vi "CreateTableSP.vi"(8 "error in (no error)":errorcluster, 10 "Name of Table":string, 11 "SimulationParameter in":refnum<class "SimulationParameter.lvclass">) -> (0 "error out":errorcluster, 1 "List of Fieldelements":string[](array[string]), 2 "Energy System Setup":string[][](table) caption="Result Set (from first statement with results)", 3 "SimulationParameter out":refnum<class "SimulationParameter.lvclass">)   [LabVIEW 2017, in "SimulationParameter.lvclass"]
uses:
  SimulationParameter.lvclass
  SimulationParameter.lvclass/SimulationParameter.ctl
  <vilib>/drjdpowell/SQLite Library/SQL Connection/Execute SQL (Single Integer).vi
  <vilib>/drjdpowell/SQLite Library/SQL Connection/Execute SQL.vi
  <vilib>/drjdpowell/SQLite Library/SQLite.lvlib
  <vilib>/drjdpowell/SQLite Library/SQL Connection/Connection.lvclass
panel:
  out "concatenated string":string
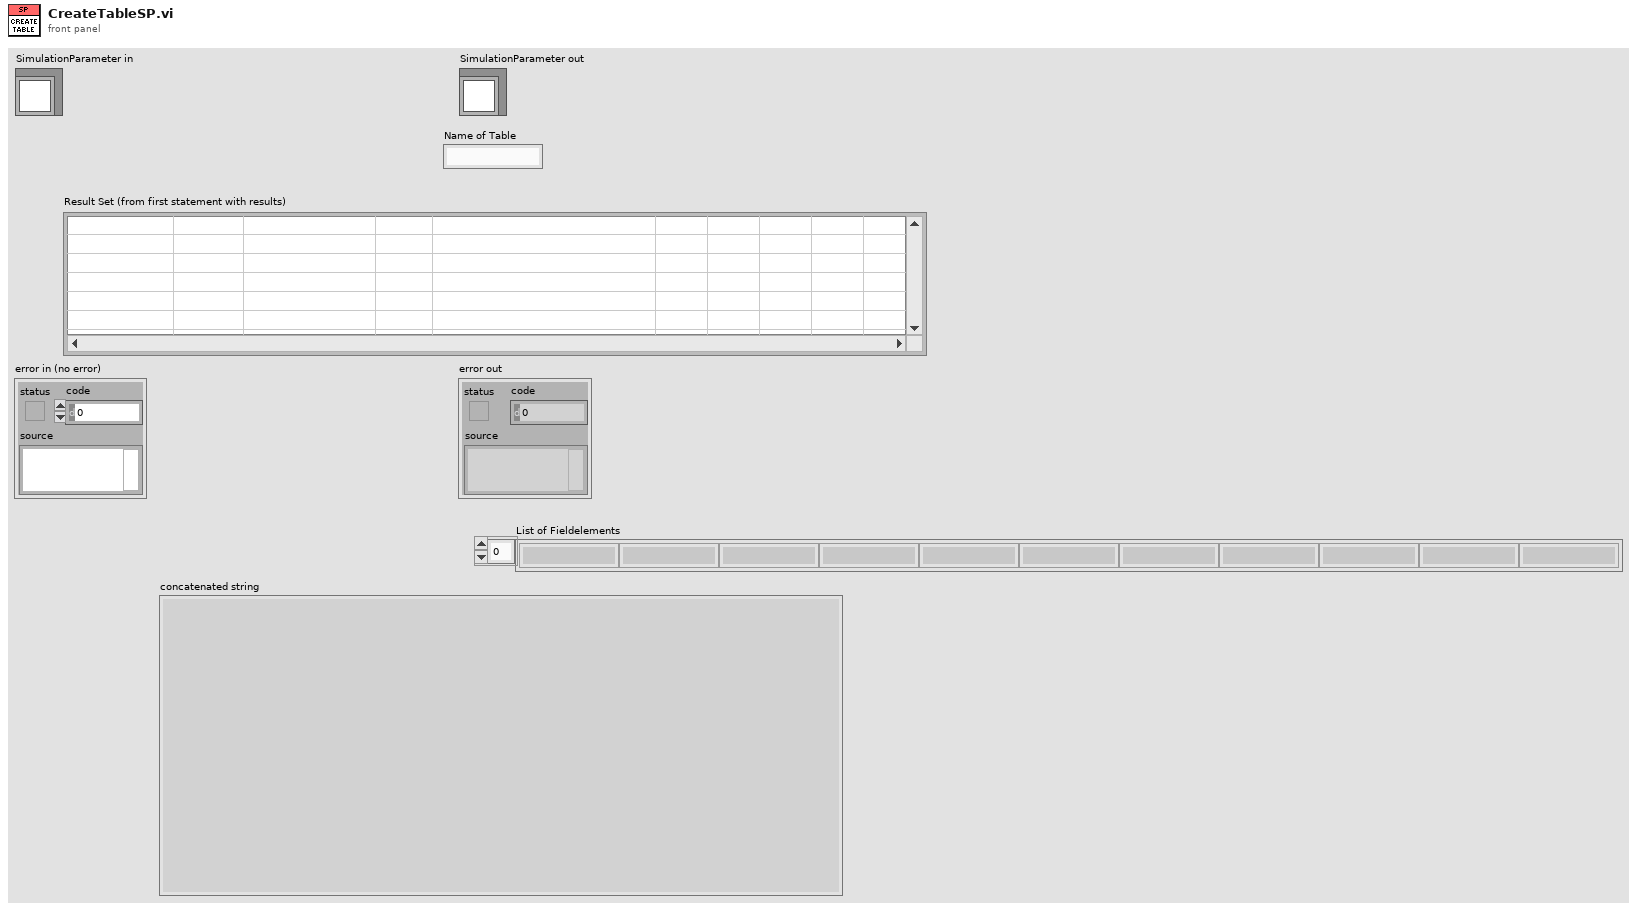
[diagram p1: front panel]
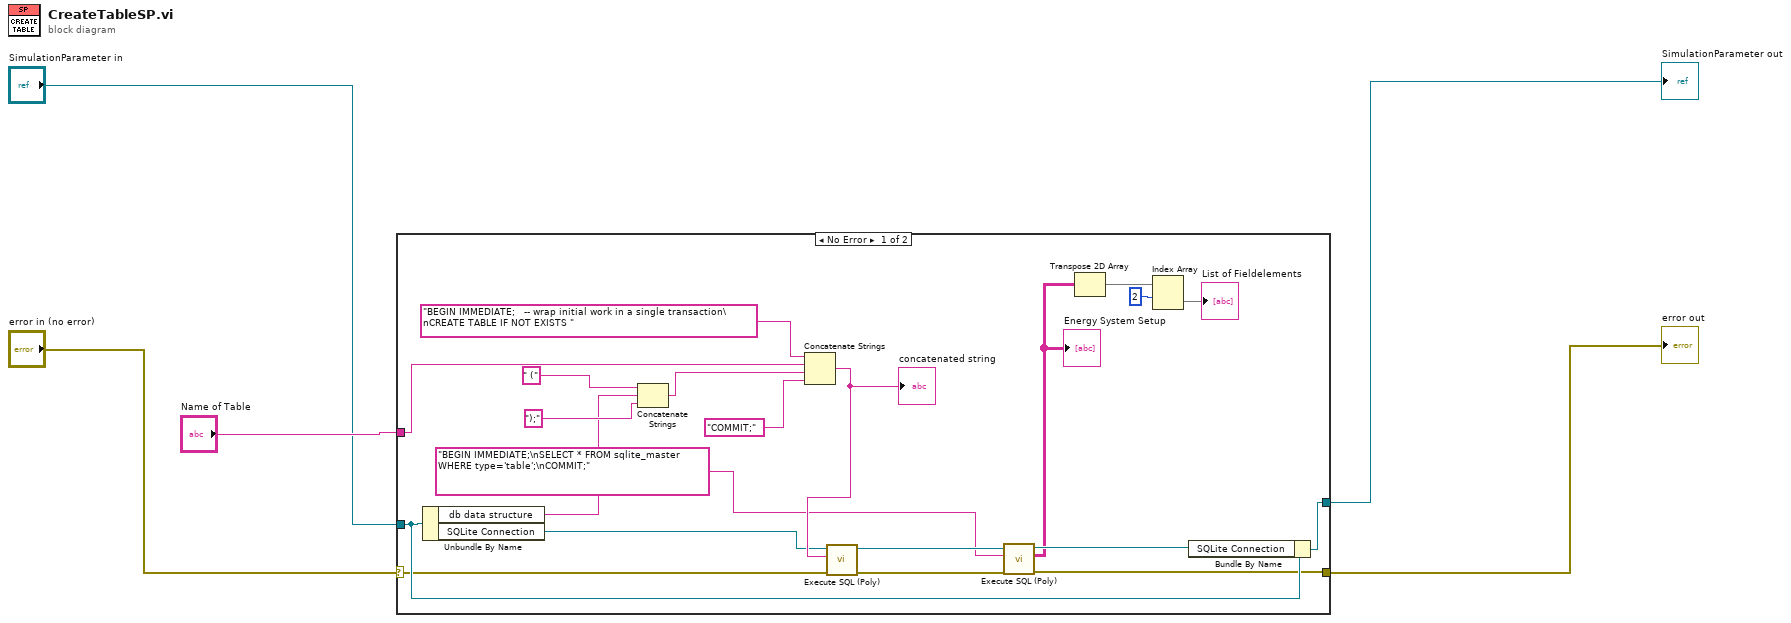
[diagram p0: block diagram]
diagram:
  n1 = case shown="No Error" "error in (no error)" {
    selector: "error in (no error)" -> [w6 w28]
    tunnel: [w9 w28] -> w2
    tunnel: [w23 w27] -> w3
    tunnel: "SimulationParameter in" -> [w22 w27]
    tunnel: "Name of Table" -> [w15 _]
    frame No Error {
      n2 = Unbundle By Name(w22) -> ("db data structure"=w14:string, "SQLite Connection"=w13:refnum<class "Connection.lvclass">)
      n3 = Concatenate Strings(" (" ("string"), w14, ");" ("string")) -> (w18:string)
      n4 = Concatenate Strings("BEGIN IMMEDIATE;   -- wrap initial work in a single transaction\nCREATE TABLE IF NOT EXISTS ", w15, w18, "COMMIT;" ("string")) -> (w19:string)
      "concatenated string" <- w19
      n5 = call-poly <vilib>:"Execute SQL (Poly).vi"("error in (no error)"=w6, "SQL"=w19, "SQLite Connection in"=w13) -> ("error out"=w10:errorcluster, "SQLite Connection out"=w12:refnum<class "Connection.lvclass">)  [unwired: 6 in, 1 out]
      n6 = call-poly <vilib>:"Execute SQL (Poly).vi"("error in (no error)"=w10, "SQL"="BEGIN IMMEDIATE;\nSELECT * FROM sqlite_master WHERE type='table';\nCOMMIT;" ("String"), "SQLite Connection in"=w12) -> ("error out"=w9:errorcluster, "Result Set"=w8:string[][], "SQLite Connection out"=w11:refnum<class "Connection.lvclass">)  [unwired: 5 in, 1 out]
      "Energy System Setup" <- w8
      n7 = Transpose 2D Array(2D array=w8) -> (transposed array=w26:string[][])
      n8 = Index Array(array=w26, index (row)=2 ("Index")) -> (element=→"List of Fieldelements":string[])  [unwired: 1 in]
      n9 = Bundle By Name(cluster=w22, "SQLite Connection"=w11) -> (w23:refnum<class "SimulationParameter.lvclass">)
    }
    frame Error {
    }
  }
  "error out" <- w2
  "SimulationParameter out" <- w3
